vi "service_sever.vi"() -> ()   [LabVIEW 2015]
uses:
  <vilib>/Tufts CEEO ROS for LabVIEW Software/ROS/MessageBuilding/std_msgs/subs/boolScalar.vi
  <vilib>/express/express shared/transition.llb/Dynamic To Waveform Array.vi
  <vilib>/express/express arith-compare/Formula/Block/exnFormulaBlock how many pts in the wave.vi
  <vilib>/express/express shared/ex_Modify Signal Name.vi
  <vilib>/express/express shared/transition.llb/Waveform Array To Dynamic.vi
  <vilib>/express/express arith-compare/Formula/XNode/ExpressFormulaBlockNode.xnode
panel:
  in  "reset":bool
  out "z":dbl
  out "y":dbl
  out "x":dbl
  in  "DO1":bool
  in  "DO4":bool
  in  "DO5":bool
  in  "DO3":bool
  in  "DO2":bool
  in  "DO0":bool
  in  "reply":bool
  in  "stop":bool
  out "Request":string
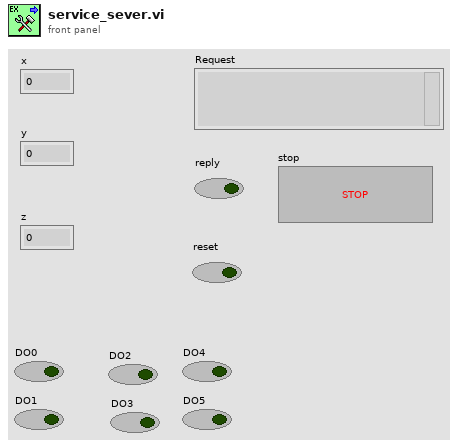
[diagram p1: front panel]
types:
  T1 = typedef "_ROSControl.ctl" = cluster{"topic port":u16, "Node":string, "topic":string, "type":string, "node port":u16, "error ":errorcluster, "Direction":T2, "Update (ms)":u16, "FIFO size":u16}
  T2 = typedef "_ROSDirection.ctl" = enum16{"Node", "Publisher", "Subscriber", "ServiceClient", "ServiceProvider"}
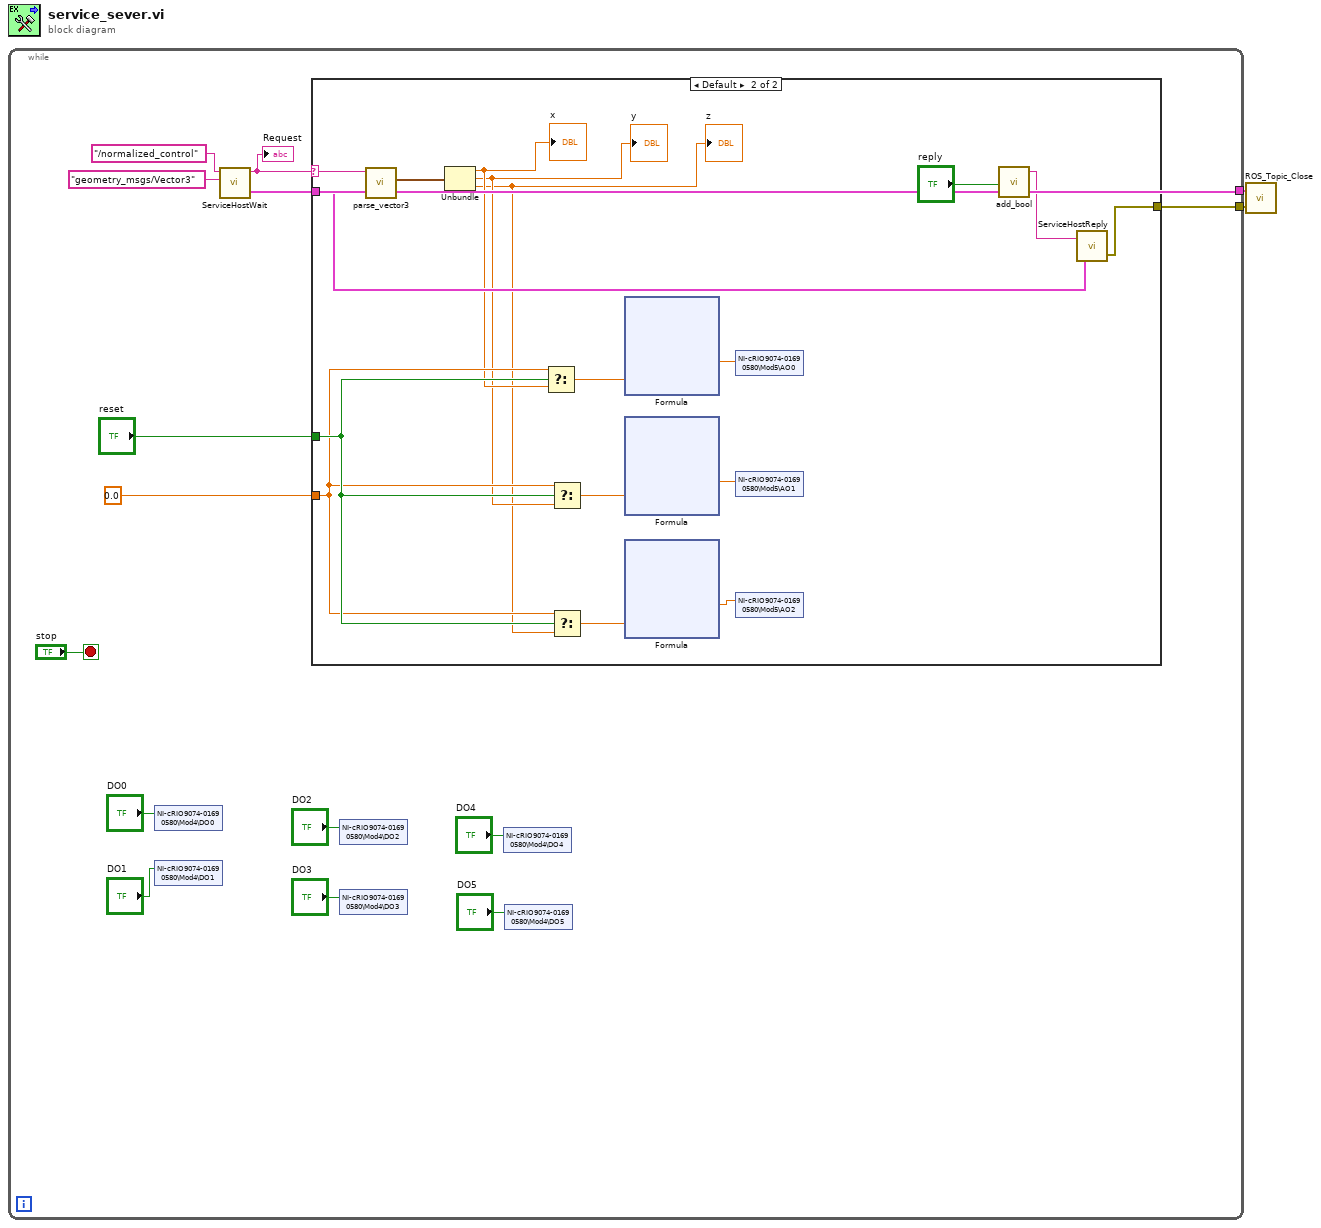
[diagram p0: block diagram]
diagram:
  n1 = while {
    tunnel: [w12] -> w2
    tunnel: [w11] -> w1
    stop <- "stop" stop-if-true
    n2 = shared-variable "NI-cRIO9074-01690580\\Mod4\\DO0"("DO0") -> ()  [unwired: 1 in, 1 out]
    n3 = shared-variable "NI-cRIO9074-01690580\\Mod4\\DO1"("DO1") -> ()  [unwired: 1 in, 1 out]
    n4 = call <userlib>:"ServiceHostWait.vi"("Topic"="/normalized_control", "Type"="geometry_msgs/Vector3") -> ("Request"=w15:string, "Service ROS info out"=w12:T1)  [unwired: 3 in]
    "Request" <- w15
    n5 = case shown="Default" w15 {
      selector: w15 -> [_ w31]
      tunnel: w12 -> [_ w33]
      tunnel: [_ w32] -> w11
      tunnel: "reset" -> [_ w24]
      tunnel: 0.0 -> [_ w23]
      frame "" {
      }
      frame Default {
        n6 = call <vilib>:"parse_vector3.vi"("msg in"=w31) -> ("Vector3"=w25:cluster{"x":dbl, "y":dbl, "z":dbl})  [unwired: 4 in, 2 out]
        n7 = Unbundle(w25) -> ("x"=w21:dbl, "y"=w20:dbl, "z"=w19:dbl)
        "x" <- w21
        "y" <- w20
        "z" <- w19
        n8 = Select(t=w23, s=w24, f=w21) -> (s? t:f=w22:dbl)
        n9 = Select(t=w23, s=w24, f=w20) -> (s? t:f=w18:dbl)
        n10 = Select(t=w23, s=w24, f=w19) -> (s? t:f=w17:dbl)
        n11 = xnode "Formula"("Pressure"=w22) -> ("Result"=w26:dbl)  [unwired: 1 in, 1 out]
        n12 = xnode "Formula"("Pressure"=w18) -> ("Result"=w28:dbl)  [unwired: 1 in, 1 out]
        n13 = xnode "Formula"("Pressure"=w17) -> ("Result"=w27:dbl)  [unwired: 1 in, 1 out]
        n14 = shared-variable "NI-cRIO9074-01690580\\Mod5\\AO0"(w26) -> ()  [unwired: 1 in, 1 out]
        n15 = shared-variable "NI-cRIO9074-01690580\\Mod5\\AO1"(w28) -> ()  [unwired: 1 in, 1 out]
        n16 = shared-variable "NI-cRIO9074-01690580\\Mod5\\AO2"(w27) -> ()  [unwired: 1 in, 1 out]
        n17 = call-poly <vilib>:"add_bool.vi"("Boolean"="reply") -> ("msg out"=w29:string)  [unwired: 4 in]
        n18 = call <userlib>:"ServiceHostReply.vi"("Service ROS info in"=w33, "Reply"=w29) -> ("error out"=w32:errorcluster)  [unwired: 2 in]
      }
    }
    n19 = shared-variable "NI-cRIO9074-01690580\\Mod4\\DO2"("DO2") -> ()  [unwired: 1 in, 1 out]
    n20 = shared-variable "NI-cRIO9074-01690580\\Mod4\\DO3"("DO3") -> ()  [unwired: 1 in, 1 out]
    n21 = shared-variable "NI-cRIO9074-01690580\\Mod4\\DO4"("DO4") -> ()  [unwired: 1 in, 1 out]
    n22 = shared-variable "NI-cRIO9074-01690580\\Mod4\\DO5"("DO5") -> ()  [unwired: 1 in, 1 out]
  }
  n23 = call <userlib>:"ROS_Topic_Close.vi"("error in"=w1, "ROS in"=w2) -> ()  [unwired: 2 in, 1 out]
